vi "ma_SML Spectrum Peak Search.vi"   [LabVIEW 2020, in "NI_MAPro.lvlib"]
uses:
  NI_MAPro.lvlib
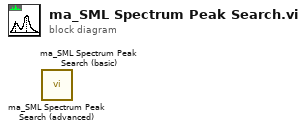
[diagram p0: block diagram]
diagram:
  n1 = call "ma_SML Spectrum Peak Search (advanced).vi"() -> ()  [unwired: 9 in, 3 out]
  n2 = call "ma_SML Spectrum Peak Search (basic).vi"() -> ()  [unwired: 9 in, 3 out]
